vi "Queue - Dequeue.vi"(8 "error in (no error)":errorcluster, 11 "Message Queue":refnum<queue>) -> (0 "error out":errorcluster, 1 "Message Data":variant, 2 "Message":string, 3 "dup Message Queue":refnum<queue>)   [LabVIEW 2024, in "QMH Messaging.lvlib"]
uses:
  QMH Messaging.lvlib
  Downloads/CLA ADAN/ATM/support/Message Queue/Message Cluster.ctl
  Downloads/CLA ADAN/ATM/support/Message Queue/Message Queue.lvlib
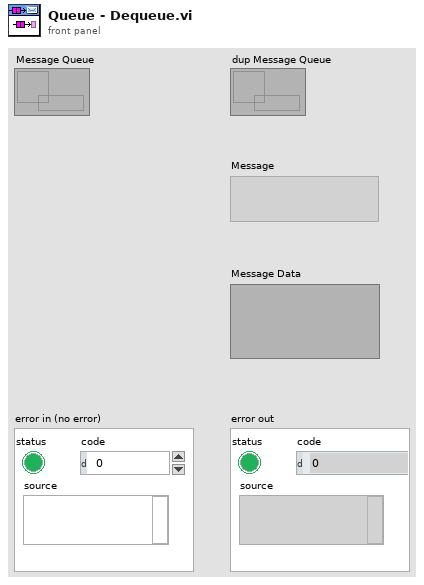
[diagram p1: front panel]
types:
  T1 = typedef "Message Queue.lvlib/Message Cluster.ctl" = cluster{"Message":string, "Message Data":variant}
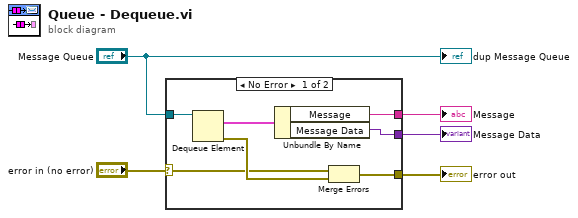
[diagram p0: block diagram]
diagram:
  n1 = case shown="No Error" "error in (no error)" {
    selector: "error in (no error)" -> [w6 w13]
    tunnel: [w11 w13] -> w5
    tunnel: [w9 _] -> w4
    tunnel: [w8 _] -> w3
    tunnel: "Message Queue" -> [w7 _]
    frame No Error {
      n2 = Dequeue Element(queue=w7) -> (element=w10:T1, error out=w12:errorcluster)  [unwired: 2 in, 2 out]
      n3 = Unbundle By Name(w10) -> ("Message"=w8:string, "Message Data"=w9:variant)
      n4 = Merge Errors(w6, w12) -> (w11:errorcluster)
    }
    frame Error {
    }
  }
  "error out" <- w5
  "Message" <- w3
  "Message Data" <- w4
  "dup Message Queue" <- "Message Queue"
